vi "Excel_Set_Chart_Scale.vi"(0 "Excel._Worksheet":refnum<k7>, 1 "gridlines":T1, 2 "Shapes":refnum<k7>, 5 "Type":i32(ring)=1 items=["xlCategory"=1, "xlSeriesAxis"=3, "xlValue"=2], 9 "Chart index":i16=-1, 11 "error in (no error)":errorcluster, 12 "axis config":T2={"autoscale"=FALSE, "min"=0.0, "max"=0.0, "scale type"=-4132} {"scale type" items=["xlScaleLinear"=-4132, "xlScaleLogarithmic"=-4133]; "max" format="%0.2f"; "min" format="%0.2f"}) -> (15 "error out":errorcluster)   [LabVIEW 2020, in "NI_ReportGenerationToolkit.lvlib"]
uses:
  <vilib>/addons/_office/NI_ReportGenerationToolkit.lvlib
panel:
  in  "Excel._OLEObject":refnum<k7>
  in  "Graph.Axes":refnum<k7>
  in  "Graph.Chart":refnum<k7>
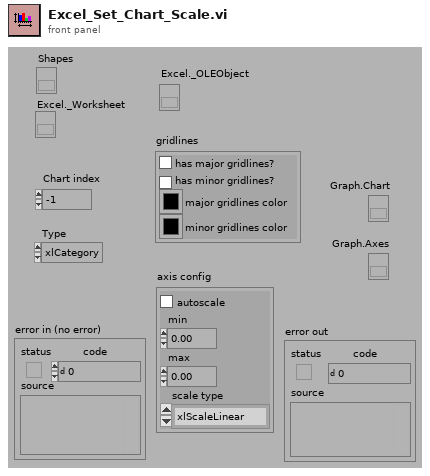
[diagram p1: front panel]
types:
  T1 = cluster{"has major gridlines?":bool, "has minor gridlines?":bool, "major gridlines color":u32, "minor gridlines color":u32}
  T2 = cluster{"autoscale":bool, "min":dbl, "max":dbl, "scale type":i32}
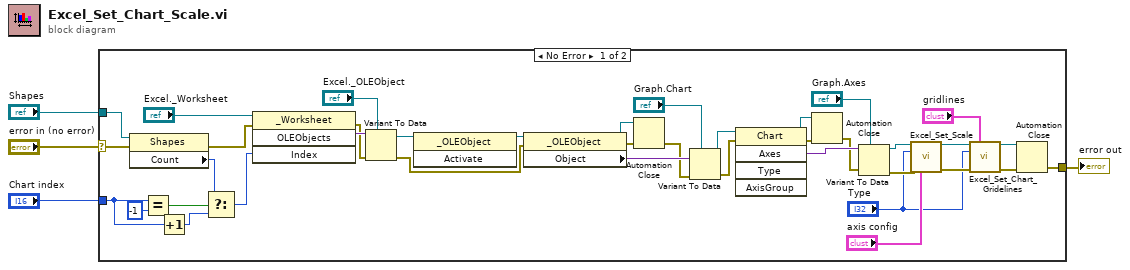
[diagram p0: block diagram]
diagram:
  n1 = case shown="No Error" "error in (no error)" {
    selector: "error in (no error)" -> [w5 w43]
    tunnel: "Chart index" -> [w20 _]
    tunnel: [w9 w43] -> w3
    tunnel: "Shapes" -> [w7 _]
    frame No Error {
      n2 = property class="Shapes"(reference=w7, error in=w5) -> (error out=w23:errorcluster, "Count"=w22:i32)  [unwired: 1 out]
      n3 = Equal?(x=w20, y=i16 -1) -> (x = y?=w31:bool)
      n4 = Increment(x=w20) -> (x+1=w29:i16)
      n5 = Select(t=w22, s=w31, f=w29) -> (s? t:f=w21:i32)
      n6 = invoke class="_Worksheet" method="OLEObjects"(reference="Excel._Worksheet", error in=w23, "Index"=w21) -> (error out=w26:errorcluster, "OLEObjects"=w27:variant)  [unwired: 1 in, 2 out]
      n7 = Variant To Data(error in=w26, type="Excel._OLEObject", Variant=w27) -> (data=w16:refnum<k7>, error out=w14:errorcluster)
      n8 = invoke class="_OLEObject" method="Activate"(reference=w16) -> (reference out=w15:refnum<k7>)  [unwired: 2 in, 2 out]
      n9 = property class="_OLEObject"(reference=w15, error in=w14) -> (reference out=w24:refnum<k7>, error out=w25:errorcluster, "Object"=w19:variant)
      n10 = Automation Close(3:w25, 5:w24) -> (0:w17:errorcluster)
      n11 = Variant To Data(error in=w17, type="Graph.Chart", Variant=w19) -> (data=w41:refnum<k7>, error out=w18:errorcluster)
      n12 = invoke class="Chart" method="Axes"(reference=w41, error in=w18) -> (reference out=w12:refnum<k7>, error out=w13:errorcluster, "Axes"=w40:variant)  [unwired: 3 in, 2 out]
      n13 = Automation Close(3:w13, 5:w12) -> (0:w36:errorcluster)
      n14 = Variant To Data(error in=w36, type="Graph.Axes", Variant=w40) -> (data=w37:refnum<k7>, error out=w38:errorcluster)
      n15 = call <vilib>:"Excel_Set_Scale.vi"("Axes in"=w37, "Type"="Type", "error in (no error)"=w38, "axis config"="axis config") -> ("Axes out"=w33:refnum<k7>, "error out"=w34:errorcluster)  [unwired: 5 in, 5 out]
      n16 = call <vilib>:"Excel_Set_Chart_Gridelines.vi"("Axes in"=w33, "gridlines"="gridlines", "Type"="Type", "error in (no error)"=w34) -> ("Axes out"=w10:refnum<k7>, "error out"=w11:errorcluster)  [unwired: 10 out]
      n17 = Automation Close(3:w11, 5:w10) -> (0:w9:errorcluster)
    }
    frame Error {
    }
  }
  "error out" <- w3
